vi "Compile Device Settings.vi"(8 "error in (no error)":errorcluster, 11 "Device Ref in":T1 format="%.0x") -> (0 "error out":errorcluster, 2 "Device Settings":T2, 3 "Device Ref out":T1 format="%.0x")   [LabVIEW 2014, in "SLSC configuration System Explorer.lvlib"]
uses:
  SLSC configuration System Explorer.lvlib
  Shared/Type Defs/Device Settings.ctl
  <vilib>/NI Veristand/Custom Device API/Custom Device Item Ref.ctl
  Shared/Constants.vi
  <vilib>/NI Veristand/Custom Device API/Get Item Property (U16).vi
  <vilib>/NI Veristand/Custom Device API/Get Item Property (U32).vi
  <vilib>/NI Veristand/Custom Device API/Get Item Property (Dependent File).vi
  <vilib>/NI Veristand/Custom Device API/Get Item Property (String).vi
  <vilib>/NI Veristand/Custom Device API/Custom Device API.lvlib
  Shared/SLSC configuration Shared.lvlib
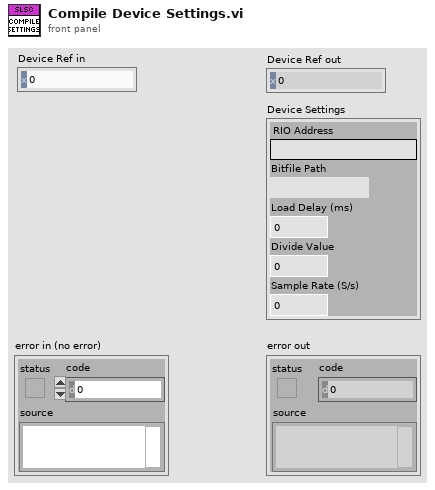
[diagram p1: front panel]
types:
  T1 = typedef "Custom Device API.lvlib/Custom Device Item Ref.ctl" = u64
  T2 = typedef "SLSC configuration Shared.lvlib/Device Settings.ctl" = cluster{"RIO Address":string, "Bitfile Path":path, "Load Delay (ms)":u32, "Divide Value":u8, "Sample Rate (S/s)":u32}
  T3 = typedef "Custom Device API.lvlib/Custom Device Target Type.ctl" = enum16{"PharLap", "VxWorks", "Windows"}
  T4 = typedef "Custom Device API.lvlib/Dependent File Optional Info.ctl" = cluster{"Version":string, "RTDestination":path, "ForceDownload":bool, "SupportedTarget":string, "MD5":string}
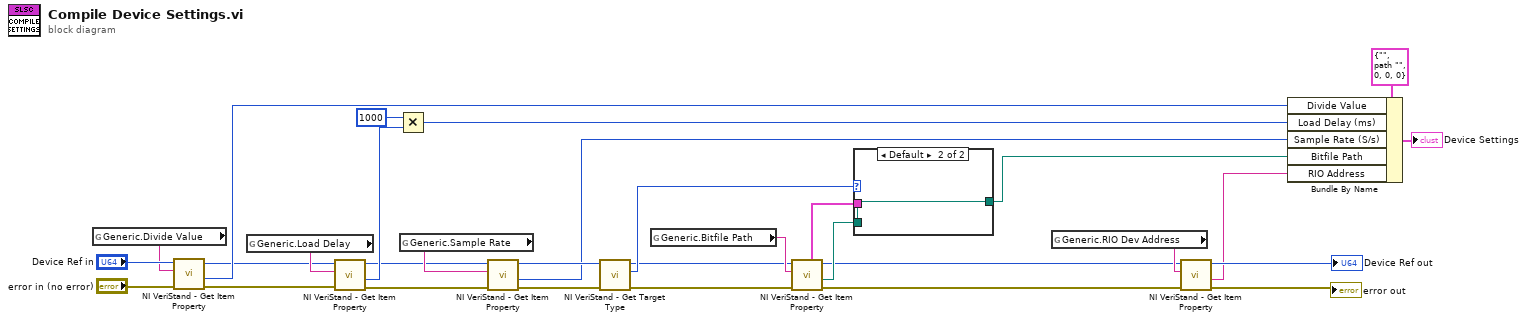
[diagram p0: block diagram]
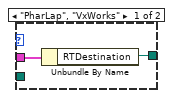
[diagram p2: hidden frame]
diagram:
  n1 = global read "Constants.vi" "Generic.Divide Value"() -> (w14:string)
  n2 = call-poly <vilib>:"NI VeriStand - Get Item Property.vi"("error in (no error)"="error in (no error)", "Property Name"=w14, "Item Ref in"="Device Ref in") -> ("error out"=w4:errorcluster, "Value"=w17:u16, "Item Ref out"=w5:T1)  [unwired: 5 in, 1 out]
  n3 = global read "Constants.vi" "Generic.Load Delay"() -> (w6:string)
  n4 = call-poly <vilib>:"NI VeriStand - Get Item Property.vi"("error in (no error)"=w4, "Property Name"=w6, "Item Ref in"=w5) -> ("error out"=w7:errorcluster, "Value"=w18:u16, "Item Ref out"=w8:T1)  [unwired: 5 in, 1 out]
  n5 = Multiply(x=u32 1000, y=w18) -> (x*y=w20:u32)
  n6 = global read "Constants.vi" "Generic.Sample Rate"() -> (w9:string)
  n7 = call-poly <vilib>:"NI VeriStand - Get Item Property.vi"("error in (no error)"=w7, "Property Name"=w9, "Item Ref in"=w8) -> ("error out"=w22:errorcluster, "Value"=w21:u32, "Item Ref out"=w23:T1)  [unwired: 5 in, 1 out]
  n8 = call <vilib>:"NI VeriStand - Get Target Type.vi"("error in (no error)"=w22, "Item Ref in"=w23) -> ("error out"=w24:errorcluster, "Target Type"=w25:T3, "Item Ref out"=w1:T1)  [unwired: 7 in]
  n9 = global read "Constants.vi" "Generic.Bitfile Path"() -> (w10:string)
  n10 = call-poly <vilib>:"NI VeriStand - Get Item Property.vi"("error in (no error)"=w24, "Property Name"=w10, "Item Ref in"=w1) -> ("error out"=w11:errorcluster, "Path"=w26:path, "Item Ref out"=w12:T1, "OptionalInfo"=w28:T4)  [unwired: 4 in, 1 out]
  n11 = case shown="Default" w25 {
    tunnel: [w32 w34] -> w27
    tunnel: w26 -> [_ w34]
    tunnel: w28 -> [w33 _]
    frame "PharLap", "VxWorks" {
      n12 = Unbundle By Name(w33) -> ("RTDestination"=w32:path)
    }
    frame Default {
    }
  }
  n13 = global read "Constants.vi" "Generic.RIO Dev Address"() -> (w13:string)
  n14 = call-poly <vilib>:"NI VeriStand - Get Item Property.vi"("error in (no error)"=w11, "Property Name"=w13, "Item Ref in"=w12) -> ("error out"=→"error out":errorcluster, "Value"=w16:string, "Item Ref out"=→"Device Ref out":T1)  [unwired: 5 in, 1 out]
  n15 = Bundle By Name(cluster=T2 {"RIO Address"="", "Bitfile Path"=path "", "Load Delay (ms)"=0, "Divide Value"=0, "Sample Rate (S/s)"=0}, "Divide Value"=w17, "Load Delay (ms)"=w20, "Sample Rate (S/s)"=w21, "Bitfile Path"=w27, "RIO Address"=w16) -> (→"Device Settings":T2)
